vi "MSEncoder SubVI pyToMSEncoder.vi"(8 "error in (no error)":errorcluster, 11 "eventProcess":string[][](array[string])) -> (0 "error out":errorcluster, 1 "Ion trap":cluster{"R0":ext, "Z0":ext}, 2 "PriRF":T1, 3 "MS ProcessFMTs":cluster{"ProcessName":string, "Data":variant}[](array[cluster]))   [LabVIEW 2018, in "MSEncoder.lvclass"]
uses:
  MSEncoder.lvclass
  Ctl/MSEditorParam header.ctl
  Ctl/MSEditorParam RFStart.ctl
  Ctl/MSEditorParam laserTrig.ctl
  Ctl/MSEditorParam ionGate.ctl
  Ctl/MSEditorParam updConj.ctl
  Ctl/MSEditorParam setDAQ.ctl
  Ctl/MSEditorParam acqSig.ctl
  Ctl/MSEditorParam wait.ctl
  Ctl/MSEditorParam updIGVolts.ctl
  Ctl/MSEditorParam updRFBias.ctl
  Ctl/MSEditorParam updRFChFunc.ctl
  Ctl/MSEditorParam resetRFCycle.ctl
  Ctl/MSEditorParam updRFScale.ctl
  Ctl/MSEditorParam updAuxArbPulses.ctl
  Ctl/MSEditorParam auxScan.ctl
  Ctl/MSEditorParam phaseScan.ctl
  Ctl/MSEditorParam phaseScanII.ctl
  Ctl/MSEditorParam linearAmpScan.ctl
  Ctl/MSEditorParam CLFreqScan.ctl
  Ctl/MSEditorParam updAO.ctl
  Ctl/MSEditorParam updDO.ctl
  Ctl/MSEditorParam FGen.ctl
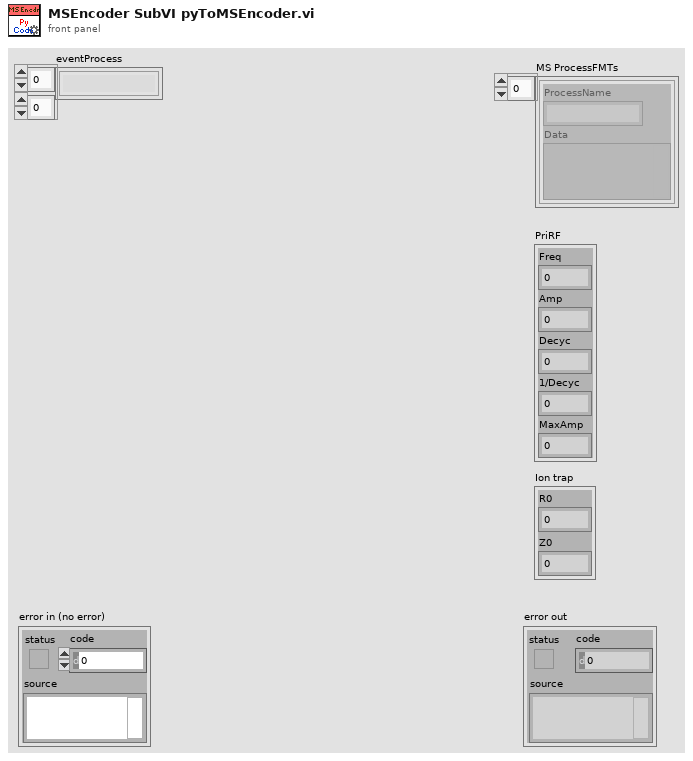
[diagram p1: front panel]
types:
  T1 = cluster{"Freq":ext, "Amp":ext, "Decyc":u32, "1/Decyc":u32, "MaxAmp":dbl}
  T2 = typedef "MSEditorParam header.ctl" = cluster{"ionTrapR0":dbl, "ionTrapZ0":dbl, "priRFMaxAmp":dbl}
  T3 = typedef "MSEditorParam RFStart.ctl" = cluster{"freq":ext, "amp":ext, "wfmType":u32}
  T4 = typedef "MSEditorParam laserTrig.ctl" = cluster{"trigFreq":ext, "phaseDeg":ext, "shots":u32}
  T5 = typedef "MSEditorParam ionGate.ctl" = cluster{"trialTime":ext, "TPH":ext, "enableAGC":bool}
  T6 = typedef "MSEditorParam updConj.ctl" = cluster{"iniPhase":u32, "conjLen":ext[], "phaseDiff":u64[], "fixedLen":bool}
  T7 = typedef "MSEditorParam setDAQ.ctl" = cluster{"channel":u32, "sampRate":u32}
  T8 = typedef "MSEditorParam acqSig.ctl" = cluster{"time ":dbl}
  T9 = typedef "MSEditorParam wait.ctl" = cluster{"timeout":ext, "DI":u16, "edge":u16}
  T10 = typedef "MSEditorParam updIGVolts.ctl" = cluster{"onVolt":dbl, "offVolt":dbl}
  T11 = typedef "MSEditorParam updRFBias.ctl" = cluster{"ch1":dbl, "ch2":dbl, "ch3":dbl}
  T12 = typedef "MSEditorParam updRFChFunc.ctl" = cluster{"ch1":u8, "ch2":u8, "ch3":u8}
  T13 = typedef "MSEditorParam resetRFCycle.ctl" = cluster{"iniPhase":u32}
  T14 = typedef "MSEditorParam updRFScale.ctl" = cluster{"ch1":dbl, "ch2":dbl, "ch3":dbl}
  T15 = typedef "MSEditorParam updAuxArbPulses.ctl" = cluster{"cycleIni":ext[], "cycleEnd":ext[], "pulseInt":ext[]}
  T16 = typedef "MSEditorParam auxScan.ctl" = cluster{"auxWfmType":u32, "auxStart":u32, "iauxCyc":ext, "auxCyc":ext[], "beta":ext[], "betaScale":ext, "auxAmp":ext[], "auxPulse1":ext[], "auxPulse2":ext[], "auxPulseAmp":ext[], "time":ext}
  T17 = typedef "MSEditorParam phaseScan.ctl" = cluster{"auxWfmType":u32, "auxStart":u32, "iauxCyc":ext, "auxCyc":ext, "beta":ext, "betaScale":ext, "auxAmp":ext, "auxPulse1":ext[], "auxPulse2":ext[], "auxPulseAmp":ext[], "time":ext, "freq":ext[], "stepWidth":u32}
  T18 = typedef "MSEditorParam phaseScanII.ctl" = cluster{"auxWfmType":u32, "auxStart":u32, "iauxCyc":ext, "auxCyc":ext, "beta":ext, "betaScale":ext, "auxAmp":ext, "auxPulse1":ext[], "auxPulse2":ext[], "auxPulseAmp":ext[], "dm":ext, "freq":ext[], "stepWidth":u32}
  T19 = typedef "MSEditorParam linearAmpScan.ctl" = cluster{"auxWfmType":u8, "iauxCyc":dbl, "beta":dbl, "betaScale":dbl, "auxAmp":ext[], "auxPulse1":dbl[], "auxPulse2":dbl[], "auxPulseAmp":ext[], "time":ext, "amp":ext[], "continuous":bool}
  T20 = typedef "MSEditorParam CLFreqScan.ctl" = cluster{"targetfreq":ext, "time":ext}
  T21 = typedef "MSEditorParam updAO.ctl" = cluster{"func":u32[], "val":ext[]}
  T22 = typedef "MSEditorParam updDO.ctl" = cluster{"func":u32[], "val":bool[]}
  T23 = typedef "MSEditorParam FGen.ctl" = cluster{"amp":ext, "freq":ext}
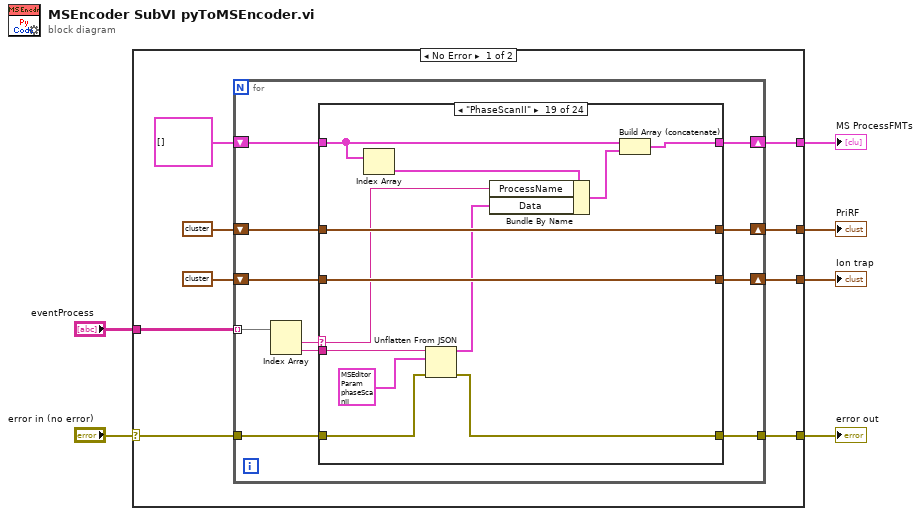
[diagram p0: block diagram]
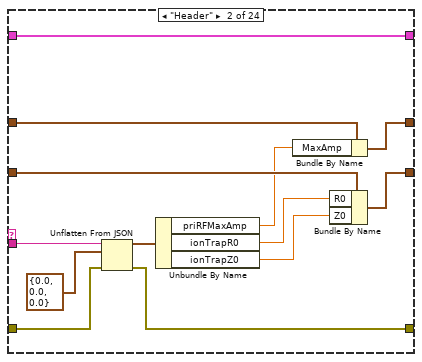
[diagram p3: hidden frame]
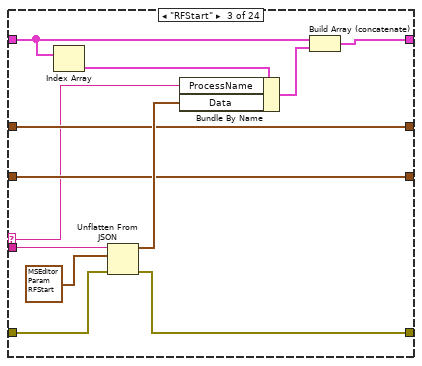
[diagram p4: hidden frame]
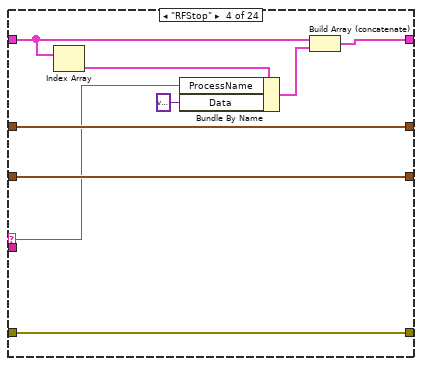
[diagram p5: hidden frame]
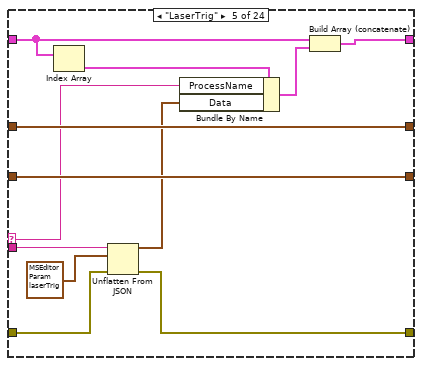
[diagram p6: hidden frame]
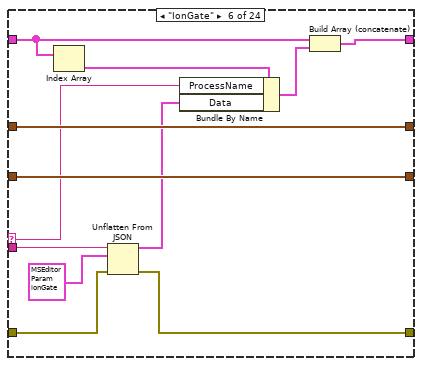
[diagram p7: hidden frame]
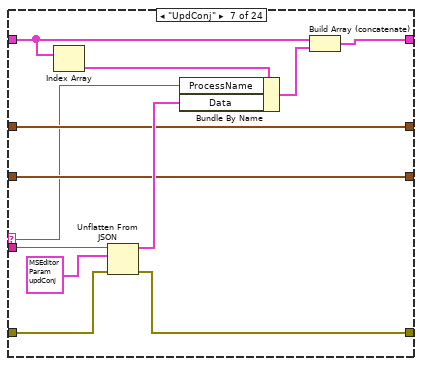
[diagram p8: hidden frame]
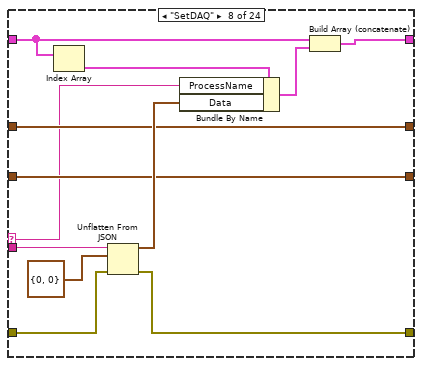
[diagram p9: hidden frame]
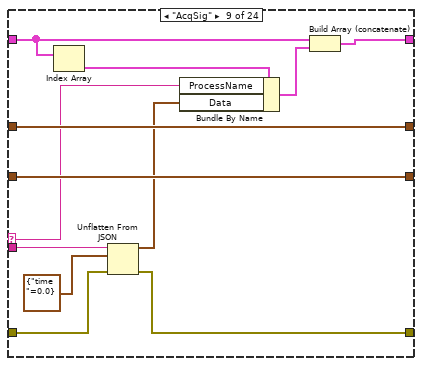
[diagram p10: hidden frame]
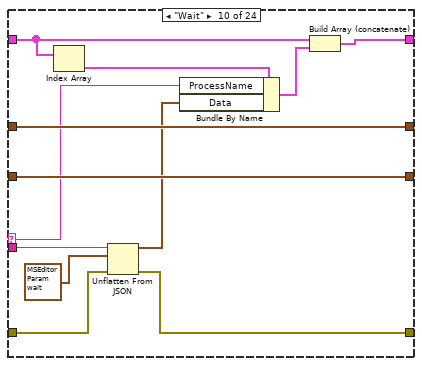
[diagram p11: hidden frame]
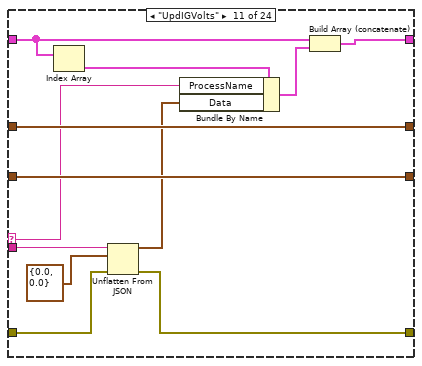
[diagram p12: hidden frame]
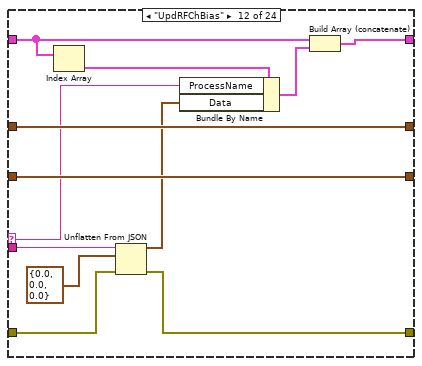
[diagram p13: hidden frame]
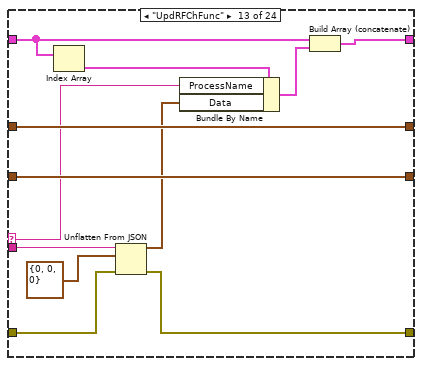
[diagram p14: hidden frame]
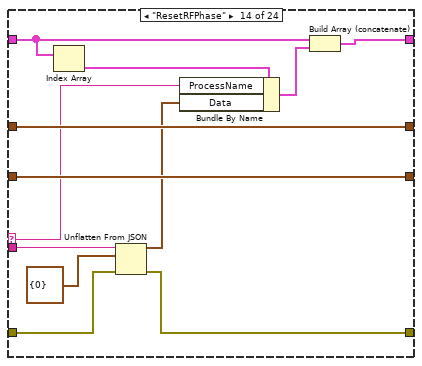
[diagram p15: hidden frame]
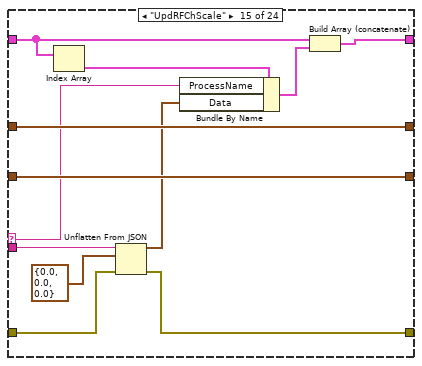
[diagram p16: hidden frame]
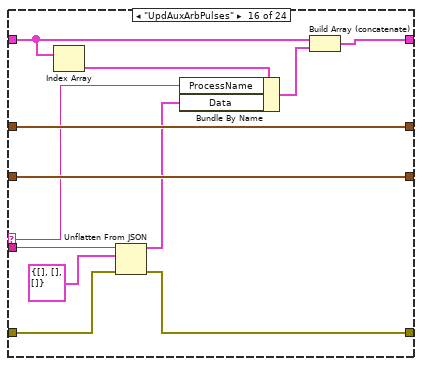
[diagram p17: hidden frame]
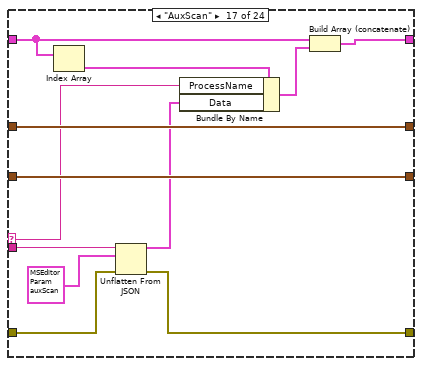
[diagram p18: hidden frame]
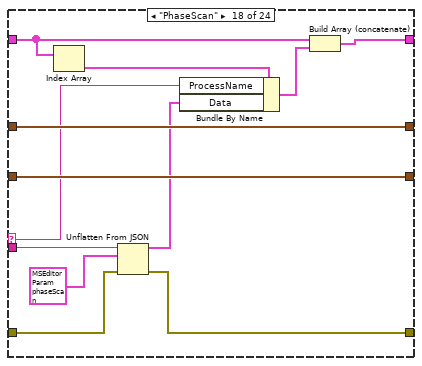
[diagram p19: hidden frame]
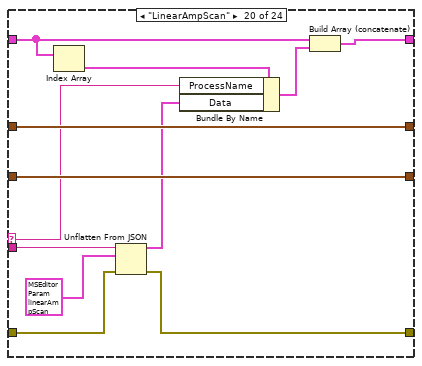
[diagram p20: hidden frame]
diagram:
  n1 = case shown="No Error" "error in (no error)" {
    selector: "error in (no error)" -> [w11 w305]
    tunnel: [w10 w305] -> w5
    tunnel: "eventProcess" -> [w15 _]
    tunnel: [w9 _] -> w3
    tunnel: [w8 _] -> w2
    tunnel: [w7 _] -> w1
    frame No Error {
      n2 = for {
        tunnel: w15 -> [w26] mode=indexing
        shift-right: [w22] -> w9
        shift-left: cluster{"ProcessName":string, "Data":variant}[] [] ("MS ProcessFMTs") -> [w23]
        tunnel: w11 -> [w19]
        tunnel: [w18] -> w10
        shift-right: [w17] -> w8
        shift-left: T1 {"Freq"=0.0, "Amp"=0.0, "Decyc"=0, "1/Decyc"=0, "MaxAmp"=0.0} ("PriRF") -> [w21]
        shift-right: [w16] -> w7
        shift-left: cluster{"R0":ext, "Z0":ext} {"R0"=0.0, "Z0"=0.0} ("Ion trap") -> [w20]
        n3 = Index Array(array=w26) -> (element #1=w25:string, element #2=w24:string)  [unwired: 2 in]
        n4 = case shown="\"PhaseScanII\"" w25 {
          selector: w25 -> [_ _ w45 w56 w67 w79 w90 w102 w115 w127 w139 w151 w163 w175 w187 w199 w211 w223 w235 w247 w259 w271 w283 w295]
          tunnel: w24 -> [_ w42 w54 _ w75 w87 w99 w111 w123 w135 w147 w159 w171 w183 w195 w207 w219 w231 w243 w255 w267 w279 w291 w303]
          tunnel: w23 -> [w30 w43 w51 w63 w73 w85 w96 w108 w121 w133 w145 w157 w169 w181 w193 w205 w217 w229 w241 w253 w265 w277 w289 w301]
          tunnel: [w30 w43 w49 w61 w71 w83 w94 w106 w119 w131 w143 w155 w167 w179 w191 w203 w215 w227 w239 w251 w263 w275 w287 w299] -> w22
          tunnel: w21 -> [w29 w38 w47 w60 w69 w81 w92 w104 w117 w129 w141 w153 w165 w177 w189 w201 w213 w225 w237 w249 w261 w273 w285 w297]
          tunnel: w20 -> [w28 w37 w46 w59 w68 w80 w91 w103 w116 w128 w140 w152 w164 w176 w188 w200 w212 w224 w236 w248 w260 w272 w284 w296]
          tunnel: w19 -> [w27 w41 w55 w57 w76 w88 w100 w112 w124 w136 w148 w160 w172 w184 w196 w208 w220 w232 w244 w256 w268 w280 w292 w304]
          tunnel: [w27 w40 w48 w57 w70 w82 w93 w105 w118 w130 w142 w154 w166 w178 w190 w202 w214 w226 w238 w250 w262 w274 w286 w298] -> w18
          tunnel: [w29 w33 w47 w60 w69 w81 w92 w104 w117 w129 w141 w153 w165 w177 w189 w201 w213 w225 w237 w249 w261 w273 w285 w297] -> w17
          tunnel: [w28 w32 w46 w59 w68 w80 w91 w103 w116 w128 w140 w152 w164 w176 w188 w200 w212 w224 w236 w248 w260 w272 w284 w296] -> w16
          frame "False", Default {
          }
          frame "Header" {
            n5 = Unflatten From JSON(JSON string=w42, type and defaults=T2 {"ionTrapR0"=0.0, "ionTrapZ0"=0.0, "priRFMaxAmp"=0.0}, error in (no error)=w41) -> (value=w39:T2, error out=w40:errorcluster)  [unwired: 4 in]
            n6 = Unbundle By Name(w39) -> ("priRFMaxAmp"=w36:dbl, "ionTrapR0"=w35:dbl, "ionTrapZ0"=w34:dbl)
            n7 = Bundle By Name(cluster=w38, "MaxAmp"=w36) -> (w33:T1)
            n8 = Bundle By Name(cluster=w37, "R0"=w35, "Z0"=w34) -> (w32:cluster{"R0":ext, "Z0":ext})
          }
          frame "RFStart" {
            n9 = Index Array(array=w51) -> (element=w53:cluster{"ProcessName":string, "Data":variant})  [unwired: 1 in]
            n10 = Unflatten From JSON(JSON string=w54, type and defaults=T3 {"freq"=0.001, "amp"=0.01, "wfmType"=0} ("ParamValueType"), error in (no error)=w55) -> (value=w52:T3, error out=w48:errorcluster)  [unwired: 4 in]
            n11 = Bundle By Name(cluster=w53, "ProcessName"=w45, "Data"=w52) -> (w50:cluster{"ProcessName":string, "Data":variant})
            n12 = Build Array (concatenate)(w51, w50) -> (w49:cluster{"ProcessName":string, "Data":variant}[])
          }
          frame "RFStop" {
            n13 = Index Array(array=w63) -> (element=w64:cluster{"ProcessName":string, "Data":variant})  [unwired: 1 in]
            n14 = Bundle By Name(cluster=w64, "ProcessName"=w56, "Data"=variant) -> (w62:cluster{"ProcessName":string, "Data":variant})
            n15 = Build Array (concatenate)(w63, w62) -> (w61:cluster{"ProcessName":string, "Data":variant}[])
          }
          frame "LaserTrig" {
            n16 = Index Array(array=w73) -> (element=w74:cluster{"ProcessName":string, "Data":variant})  [unwired: 1 in]
            n17 = Unflatten From JSON(JSON string=w75, type and defaults=T4 {"trigFreq"=100.0, "phaseDeg"=90.0, "shots"=1} ("ParamValueType"), error in (no error)=w76) -> (value=w66:T4, error out=w70:errorcluster)  [unwired: 4 in]
            n18 = Bundle By Name(cluster=w74, "ProcessName"=w67, "Data"=w66) -> (w72:cluster{"ProcessName":string, "Data":variant})
            n19 = Build Array (concatenate)(w73, w72) -> (w71:cluster{"ProcessName":string, "Data":variant}[])
          }
          frame "IonGate" {
            n20 = Index Array(array=w85) -> (element=w86:cluster{"ProcessName":string, "Data":variant})  [unwired: 1 in]
            n21 = Unflatten From JSON(JSON string=w87, type and defaults=T5 {"trialTime"=0.1, "TPH"=1.0, "enableAGC"=FALSE} ("ParamValueType"), error in (no error)=w88) -> (value=w78:T5, error out=w82:errorcluster)  [unwired: 4 in]
            n22 = Bundle By Name(cluster=w86, "ProcessName"=w79, "Data"=w78) -> (w84:cluster{"ProcessName":string, "Data":variant})
            n23 = Build Array (concatenate)(w85, w84) -> (w83:cluster{"ProcessName":string, "Data":variant}[])
          }
          frame "UpdConj" {
            n24 = Index Array(array=w96) -> (element=w98:cluster{"ProcessName":string, "Data":variant})  [unwired: 1 in]
            n25 = Unflatten From JSON(JSON string=w99, type and defaults=T6 {"iniPhase"=2147483648, "conjLen"=[3.0, 3.0], "phaseDiff"=[2147483648, 2147483648], "fixedLen"=FALSE} ("ParamValueType"), error in (no error)=w100) -> (value=w97:T6, error out=w93:errorcluster)  [unwired: 4 in]
            n26 = Bundle By Name(cluster=w98, "ProcessName"=w90, "Data"=w97) -> (w95:cluster{"ProcessName":string, "Data":variant})
            n27 = Build Array (concatenate)(w96, w95) -> (w94:cluster{"ProcessName":string, "Data":variant}[])
          }
          frame "SetDAQ" {
            n28 = Index Array(array=w108) -> (element=w110:cluster{"ProcessName":string, "Data":variant})  [unwired: 1 in]
            n29 = Unflatten From JSON(JSON string=w111, type and defaults=T7 {"channel"=0, "sampRate"=0} ("ParamValueType"), error in (no error)=w112) -> (value=w109:T7, error out=w105:errorcluster)  [unwired: 4 in]
            n30 = Bundle By Name(cluster=w110, "ProcessName"=w102, "Data"=w109) -> (w107:cluster{"ProcessName":string, "Data":variant})
            n31 = Build Array (concatenate)(w108, w107) -> (w106:cluster{"ProcessName":string, "Data":variant}[])
          }
          frame "AcqSig" {
            n32 = Index Array(array=w121) -> (element=w122:cluster{"ProcessName":string, "Data":variant})  [unwired: 1 in]
            n33 = Unflatten From JSON(JSON string=w123, type and defaults=T8 {"time "=0.0} ("ParamValueType"), error in (no error)=w124) -> (value=w114:T8, error out=w118:errorcluster)  [unwired: 4 in]
            n34 = Bundle By Name(cluster=w122, "ProcessName"=w115, "Data"=w114) -> (w120:cluster{"ProcessName":string, "Data":variant})
            n35 = Build Array (concatenate)(w121, w120) -> (w119:cluster{"ProcessName":string, "Data":variant}[])
          }
          frame "Wait" {
            n36 = Index Array(array=w133) -> (element=w134:cluster{"ProcessName":string, "Data":variant})  [unwired: 1 in]
            n37 = Unflatten From JSON(JSON string=w135, type and defaults=T9 {"timeout"=0.001, "DI"=0, "edge"=0} ("ParamValueType"), error in (no error)=w136) -> (value=w126:T9, error out=w130:errorcluster)  [unwired: 4 in]
            n38 = Bundle By Name(cluster=w134, "ProcessName"=w127, "Data"=w126) -> (w132:cluster{"ProcessName":string, "Data":variant})
            n39 = Build Array (concatenate)(w133, w132) -> (w131:cluster{"ProcessName":string, "Data":variant}[])
          }
          frame "UpdIGVolts" {
            n40 = Index Array(array=w145) -> (element=w146:cluster{"ProcessName":string, "Data":variant})  [unwired: 1 in]
            n41 = Unflatten From JSON(JSON string=w147, type and defaults=T10 {"onVolt"=0.0, "offVolt"=0.0} ("ParamValueType"), error in (no error)=w148) -> (value=w138:T10, error out=w142:errorcluster)  [unwired: 4 in]
            n42 = Bundle By Name(cluster=w146, "ProcessName"=w139, "Data"=w138) -> (w144:cluster{"ProcessName":string, "Data":variant})
            n43 = Build Array (concatenate)(w145, w144) -> (w143:cluster{"ProcessName":string, "Data":variant}[])
          }
          frame "UpdRFChBias" {
            n44 = Index Array(array=w157) -> (element=w158:cluster{"ProcessName":string, "Data":variant})  [unwired: 1 in]
            n45 = Unflatten From JSON(JSON string=w159, type and defaults=T11 {"ch1"=0.0, "ch2"=0.0, "ch3"=0.0} ("ParamValueType"), error in (no error)=w160) -> (value=w150:T11, error out=w154:errorcluster)  [unwired: 4 in]
            n46 = Bundle By Name(cluster=w158, "ProcessName"=w151, "Data"=w150) -> (w156:cluster{"ProcessName":string, "Data":variant})
            n47 = Build Array (concatenate)(w157, w156) -> (w155:cluster{"ProcessName":string, "Data":variant}[])
          }
          frame "UpdRFChFunc" {
            n48 = Index Array(array=w169) -> (element=w170:cluster{"ProcessName":string, "Data":variant})  [unwired: 1 in]
            n49 = Unflatten From JSON(JSON string=w171, type and defaults=T12 {"ch1"=0, "ch2"=0, "ch3"=0} ("ParamValueType"), error in (no error)=w172) -> (value=w162:T12, error out=w166:errorcluster)  [unwired: 4 in]
            n50 = Bundle By Name(cluster=w170, "ProcessName"=w163, "Data"=w162) -> (w168:cluster{"ProcessName":string, "Data":variant})
            n51 = Build Array (concatenate)(w169, w168) -> (w167:cluster{"ProcessName":string, "Data":variant}[])
          }
          frame "ResetRFPhase" {
            n52 = Index Array(array=w181) -> (element=w182:cluster{"ProcessName":string, "Data":variant})  [unwired: 1 in]
            n53 = Unflatten From JSON(JSON string=w183, type and defaults=T13 {"iniPhase"=0} ("ParamValueType"), error in (no error)=w184) -> (value=w174:T13, error out=w178:errorcluster)  [unwired: 4 in]
            n54 = Bundle By Name(cluster=w182, "ProcessName"=w175, "Data"=w174) -> (w180:cluster{"ProcessName":string, "Data":variant})
            n55 = Build Array (concatenate)(w181, w180) -> (w179:cluster{"ProcessName":string, "Data":variant}[])
          }
          frame "UpdRFChScale" {
            n56 = Index Array(array=w193) -> (element=w194:cluster{"ProcessName":string, "Data":variant})  [unwired: 1 in]
            n57 = Unflatten From JSON(JSON string=w195, type and defaults=T14 {"ch1"=0.0, "ch2"=0.0, "ch3"=0.0} ("ParamValueType"), error in (no error)=w196) -> (value=w186:T14, error out=w190:errorcluster)  [unwired: 4 in]
            n58 = Bundle By Name(cluster=w194, "ProcessName"=w187, "Data"=w186) -> (w192:cluster{"ProcessName":string, "Data":variant})
            n59 = Build Array (concatenate)(w193, w192) -> (w191:cluster{"ProcessName":string, "Data":variant}[])
          }
          frame "UpdAuxArbPulses" {
            n60 = Index Array(array=w205) -> (element=w206:cluster{"ProcessName":string, "Data":variant})  [unwired: 1 in]
            n61 = Unflatten From JSON(JSON string=w207, type and defaults=T15 {"cycleIni"=[], "cycleEnd"=[], "pulseInt"=[]} ("Param"), error in (no error)=w208) -> (value=w198:T15, error out=w202:errorcluster)  [unwired: 4 in]
            n62 = Bundle By Name(cluster=w206, "ProcessName"=w199, "Data"=w198) -> (w204:cluster{"ProcessName":string, "Data":variant})
            n63 = Build Array (concatenate)(w205, w204) -> (w203:cluster{"ProcessName":string, "Data":variant}[])
          }
          frame "AuxScan" {
            n64 = Index Array(array=w217) -> (element=w218:cluster{"ProcessName":string, "Data":variant})  [unwired: 1 in]
            n65 = Unflatten From JSON(JSON string=w219, type and defaults=T16 {"auxWfmType"=0, "auxStart"=0, "iauxCyc"=0.0, "auxCyc"=[1.0, 1.0], "beta"=[0.1, 0.5], "betaScale"=1.0, "auxAmp"=[1.0, 1.0], "auxPulse1"=[0.0, 0.5], "auxPulse2"=[0.5, 1.0], "auxPulseAmp"=[1.0, -1.0], "time"=1.0} ("ParamValueType"), error in (no error)=w220) -> (value=w210:T16, error out=w214:errorcluster)  [unwired: 4 in]
            n66 = Bundle By Name(cluster=w218, "ProcessName"=w211, "Data"=w210) -> (w216:cluster{"ProcessName":string, "Data":variant})
            n67 = Build Array (concatenate)(w217, w216) -> (w215:cluster{"ProcessName":string, "Data":variant}[])
          }
          frame "PhaseScan" {
            n68 = Index Array(array=w229) -> (element=w230:cluster{"ProcessName":string, "Data":variant})  [unwired: 1 in]
            n69 = Unflatten From JSON(JSON string=w231, type and defaults=T17 {"auxWfmType"=0, "auxStart"=0, "iauxCyc"=0.0, "auxCyc"=0.0, "beta"=0.5, "betaScale"=1.0, "auxAmp"=1.0, "auxPulse1"=[0.0, 0.5], "auxPulse2"=[0.5, 1.0], "auxPulseAmp"=[1.0, -1.0], "time"=1.0, "freq"=[100000.0, 50000.0], "stepWidth"=1} ("ParamValueType"), error in (no error)=w232) -> (value=w222:T17, error out=w226:errorcluster)  [unwired: 4 in]
            n70 = Bundle By Name(cluster=w230, "ProcessName"=w223, "Data"=w222) -> (w228:cluster{"ProcessName":string, "Data":variant})
            n71 = Build Array (concatenate)(w229, w228) -> (w227:cluster{"ProcessName":string, "Data":variant}[])
          }
          frame "PhaseScanII" {
            n72 = Index Array(array=w241) -> (element=w242:cluster{"ProcessName":string, "Data":variant})  [unwired: 1 in]
            n73 = Unflatten From JSON(JSON string=w243, type and defaults=T18 {"auxWfmType"=0, "auxStart"=0, "iauxCyc"=0.0, "auxCyc"=0.0, "beta"=0.5, "betaScale"=1.0, "auxAmp"=1.0, "auxPulse1"=[0.0, 0.5], "auxPulse2"=[0.5, 1.0], "auxPulseAmp"=[1.0, -1.0], "dm"=1.0, "freq"=[100000.0, 50000.0], "stepWidth"=1} ("ParamValueType"), error in (no error)=w244) -> (value=w234:T18, error out=w238:errorcluster)  [unwired: 4 in]
            n74 = Bundle By Name(cluster=w242, "ProcessName"=w235, "Data"=w234) -> (w240:cluster{"ProcessName":string, "Data":variant})
            n75 = Build Array (concatenate)(w241, w240) -> (w239:cluster{"ProcessName":string, "Data":variant}[])
          }
          frame "LinearAmpScan" {
            n76 = Index Array(array=w253) -> (element=w254:cluster{"ProcessName":string, "Data":variant})  [unwired: 1 in]
            n77 = Unflatten From JSON(JSON string=w255, type and defaults=T19 {"auxWfmType"=0, "iauxCyc"=0.0, "beta"=0.0, "betaScale"=0.0, "auxAmp"=[], "auxPulse1"=[], "auxPulse2"=[], "auxPulseAmp"=[], "time"=0.0, "amp"=[], "continuous"=FALSE}, error in (no error)=w256) -> (value=w246:T19, error out=w250:errorcluster)  [unwired: 4 in]
            n78 = Bundle By Name(cluster=w254, "ProcessName"=w247, "Data"=w246) -> (w252:cluster{"ProcessName":string, "Data":variant})
            n79 = Build Array (concatenate)(w253, w252) -> (w251:cluster{"ProcessName":string, "Data":variant}[])
          }
          frame "CLFreqScan" {
            n80 = Index Array(array=w265) -> (element=w266:cluster{"ProcessName":string, "Data":variant})  [unwired: 1 in]
            n81 = Unflatten From JSON(JSON string=w267, type and defaults=T20 {"targetfreq"=1.0, "time"=1.0} ("clFreqScan"), error in (no error)=w268) -> (value=w258:T20, error out=w262:errorcluster)  [unwired: 4 in]
            n82 = Bundle By Name(cluster=w266, "ProcessName"=w259, "Data"=w258) -> (w264:cluster{"ProcessName":string, "Data":variant})
            n83 = Build Array (concatenate)(w265, w264) -> (w263:cluster{"ProcessName":string, "Data":variant}[])
          }
          frame "UpdAO" {
            n84 = Index Array(array=w277) -> (element=w278:cluster{"ProcessName":string, "Data":variant})  [unwired: 1 in]
            n85 = Unflatten From JSON(JSON string=w279, type and defaults=T21 {"func"=[0, 0, 0, 0], "val"=[0.0, 0.0, 0.0, 0.0]} ("updAO"), error in (no error)=w280) -> (value=w270:T21, error out=w274:errorcluster)  [unwired: 4 in]
            n86 = Bundle By Name(cluster=w278, "ProcessName"=w271, "Data"=w270) -> (w276:cluster{"ProcessName":string, "Data":variant})
            n87 = Build Array (concatenate)(w277, w276) -> (w275:cluster{"ProcessName":string, "Data":variant}[])
          }
          frame "UpdDO" {
            n88 = Index Array(array=w289) -> (element=w290:cluster{"ProcessName":string, "Data":variant})  [unwired: 1 in]
            n89 = Unflatten From JSON(JSON string=w291, type and defaults=T22 {"func"=[1, 2, 0, 0], "val"=[FALSE, FALSE, FALSE, FALSE]} ("updDO"), error in (no error)=w292) -> (value=w282:T22, error out=w286:errorcluster)  [unwired: 4 in]
            n90 = Bundle By Name(cluster=w290, "ProcessName"=w283, "Data"=w282) -> (w288:cluster{"ProcessName":string, "Data":variant})
            n91 = Build Array (concatenate)(w289, w288) -> (w287:cluster{"ProcessName":string, "Data":variant}[])
          }
          frame "UpdFGen" {
            n92 = Index Array(array=w301) -> (element=w302:cluster{"ProcessName":string, "Data":variant})  [unwired: 1 in]
            n93 = Unflatten From JSON(JSON string=w303, type and defaults=T23 {"amp"=0.001, "freq"=0.01} ("FGen"), error in (no error)=w304) -> (value=w294:T23, error out=w298:errorcluster)  [unwired: 4 in]
            n94 = Bundle By Name(cluster=w302, "ProcessName"=w295, "Data"=w294) -> (w300:cluster{"ProcessName":string, "Data":variant})
            n95 = Build Array (concatenate)(w301, w300) -> (w299:cluster{"ProcessName":string, "Data":variant}[])
          }
        }
      }
    }
    frame Error {
    }
  }
  "error out" <- w5
  "Ion trap" <- w1
  "PriRF" <- w2
  "MS ProcessFMTs" <- w3
